vi "Set_Hi-Tec_server.vi"(4 "Client Name":string, 6 "Density Ratio":string, 7 "Strength (% by volume)":dbl min=0.0 max=5.0 format="%.3f", 8 "Stack flowrate (l/min)":dbl format="%.2f", 9 "Mode":enum16{"Control Hi-Tec", "Check Hi-Tec Demands"}(ring)) -> (0 "Flowrates (kg/min)":dbl[](array[numeric]) format="%.2f", 1 "Comment":string)   [LabVIEW 2012]
uses:
  ADAM Client/Sub VIs/ADAM Controls/Update_scan_value.ctl
  ADAM Client/Sub VIs/ADAM Controls/Ch_description_ADAM.ctl
  ADAM Client/Sub VIs/ADAM Controls/Module_type_ADAM.ctl
  ADAM Client/Sub VIs/ADAM Controls/Function_ADAM.ctl
  ADAM Client/Sub VIs/ADAM Controls/Channel_State.ctl
  ADAM Client/Sub VIs/ADAM Controls/Calib_type_ADAM.ctl
  ADAM Client/Sub VIs/ADAM Controls/Address.ctl
  Anemometry/Anemometry Sub Vis/Globals/Gas_management_global.vi
panel:
  # "-Carrier 1 only\n-Carrier 2 only\n-Enter Ratio"
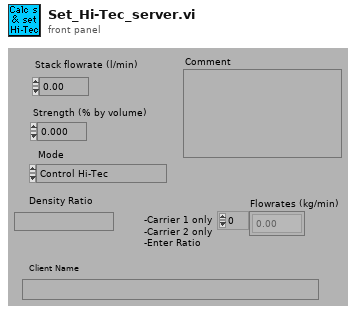
[diagram p1: front panel]
types:
  T1 = enum16{"Append to Global", "Read Global then Clear"}
  T2 = typedef "Calib_type_ADAM.ctl" = enum16{"Raw", "Bx + A", "Cx^2 + Bx + A", "Dx^3 + Cx^2 + Bx + A", "In Band", "Hi-Tec Q", "Hi-Tec M_dot", "Text"}
  T3 = typedef "Module_type_ADAM.ctl" = string
  T4 = typedef "Update_scan_value.ctl" = cluster{"Channel Name":string, "New Value":dbl}
  T5 = typedef "Ch_description_ADAM.ctl" = cluster{"Ch Name":string, "Type":T3, "Function":T6, "Ch State":T7, "Calibration type":T2, "A":dbl, "B":dbl, "C":dbl, "D":dbl, "Comments":string, "Address":T8, "String":string, "Duty":u16}
  T6 = typedef "Function_ADAM.ctl" = enum16{"Analogue Input", "Digital Input", "Event counter", "Event rate", "Analogue Output", "Digital Output", "Relay Output"}
  T7 = typedef "Channel_State.ctl" = enum16{"On", "Off", "Always On", "Always Off"}
  T8 = typedef "Address.ctl" = cluster{"Main":i32, "Ch.":i32, "Sub":i32, "Port Name":string}
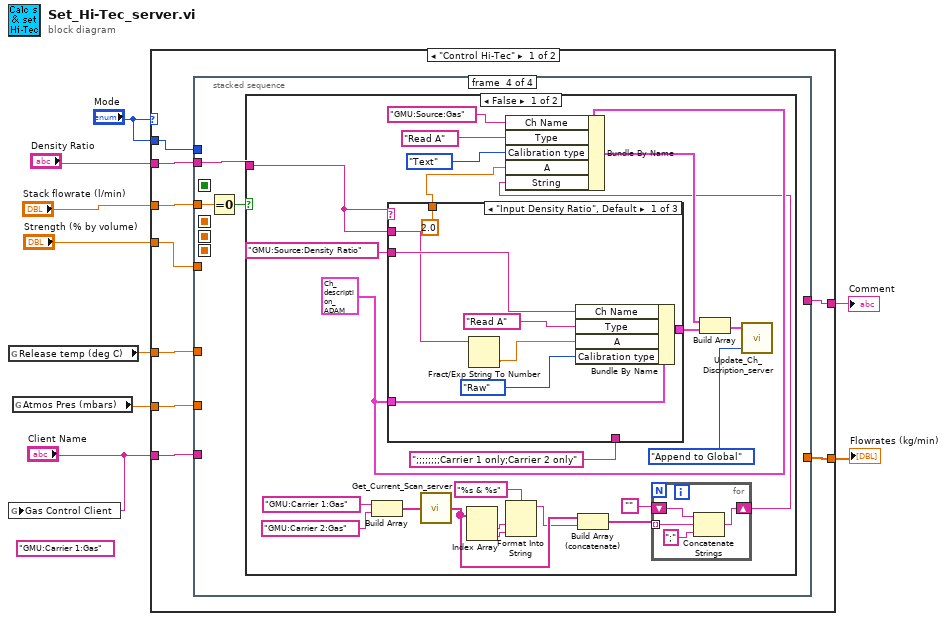
[diagram p0: block diagram]
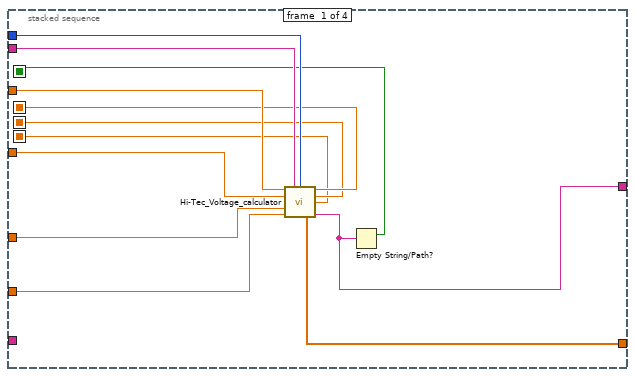
[diagram p2: hidden frame]
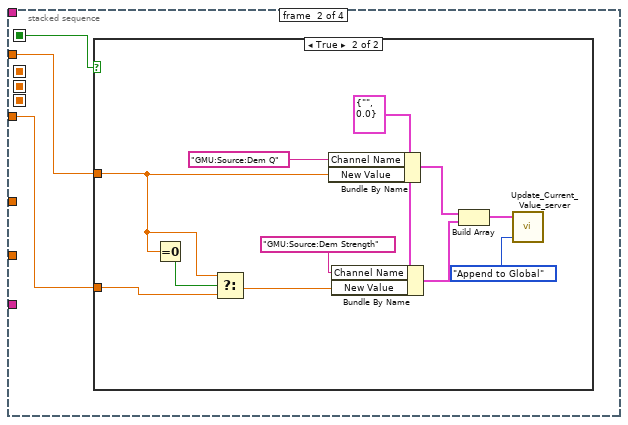
[diagram p3: hidden frame]
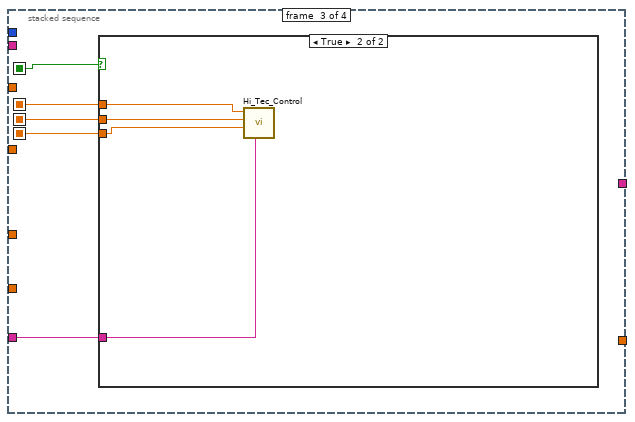
[diagram p5: hidden frame]
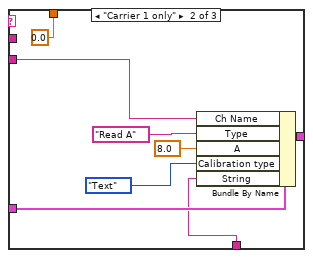
[diagram p7: hidden frame]
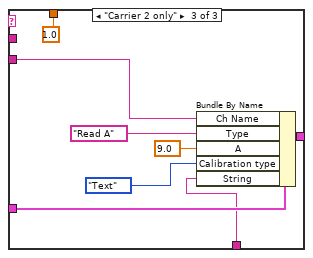
[diagram p8: hidden frame]
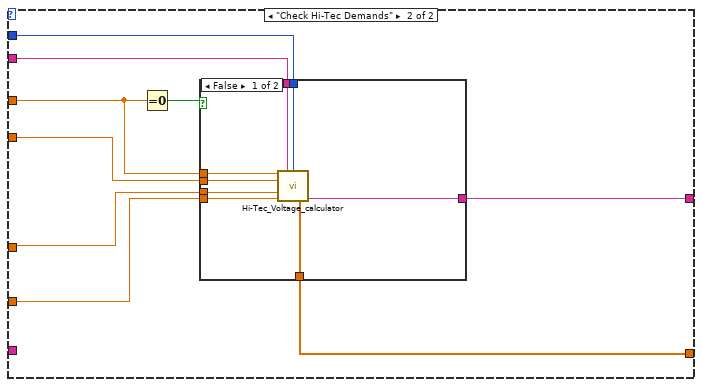
[diagram p10: hidden frame]
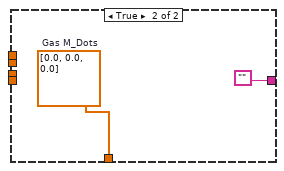
[diagram p11: hidden frame]
diagram:
  (unwired) "GMU:Carrier 1:Gas"
  n1 = global read "Gas_management_global.vi" "Release temp (deg C)"() -> (w5:dbl)
  n2 = global write "Gas_management_global.vi" "Gas Control Client"("Client Name") -> ()
  n3 = global read "Gas_management_global.vi" "Atmos Pres (mbars)"() -> (w7:dbl)
  n4 = case shown="\"Control Hi-Tec\"" "Mode" {
    tunnel: "Density Ratio" -> [w18 w113]
    tunnel: "Strength (% by volume)" -> [w17 w116]
    tunnel: "Stack flowrate (l/min)" -> [w16 w111]
    tunnel: w5 -> [w15 w115]
    tunnel: w7 -> [w14 w114]
    tunnel: [w13 w112] -> w6
    tunnel: [w12 w109] -> w3
    tunnel: "Mode" -> [w11 w108]
    tunnel: "Client Name" -> [w10 _]
    frame "Control Hi-Tec" {
      n5 = stacked-sequence {
        seq-local: [w22 _ _ _] -> [_ w31 w45 _]
        seq-local: [w21 _ _ _] -> [_ _ w49 _]
        seq-local: [w20 _ _ _] -> [_ _ w48 _]
        seq-local: [w19 _ _ _] -> [_ _ w47 _]
        tunnel: w18 -> [w28 _ _ w56]
        tunnel: w17 -> [w27 w32 _ _]
        tunnel: w16 -> [w26 w33 _ w55]
        tunnel: w15 -> [w30 _ _ _]
        tunnel: w14 -> [w29 _ _ _]
        tunnel: [w23 _ _ _] -> w13
        tunnel: [w25 _ _ _] -> w12
        tunnel: w11 -> [w24 _ _ _]
        tunnel: w10 -> [_ _ w46 _]
        frame #0 {
          n6 = call "Hi-Tec_Voltage_calculator.vi"("Stack Flowrate (l/min)"=w26, "Density Ratio"=w28, "Mode"=w24, "Strength (% by volume)"=w27, "Release temp (deg C)"=w30, "Atmos Pres (mbars)"=w29) -> ("Carrier 1 Voltage"=w21:dbl, "Carrier 2 Voltage"=w20:dbl, "Trace Voltage"=w19:dbl, "Flowrates (kg/min)"=w25:dbl[], "Error Comments"=w23:string)  [unwired: 2 in, 3 out]
          n7 = Empty String/Path?(string/path=w23) -> (empty?=w22:bool)
        }
        frame #1 {
          n8 = case shown="True" w31 {
            tunnel: w33 -> [_ w44]
            tunnel: w32 -> [_ w43]
            frame False {
            }
            frame True {
              w38 = T4 {"Channel Name"="", "New Value"=0.0} ("Update Scan Value Cluster")
              n9 = Equal To 0?(x=w44) -> (x = 0?=w35:bool)
              n10 = Select(t=w44, s=w35, f=w43) -> (s? t:f=w34:dbl)
              n11 = Bundle By Name(cluster=w38, "Channel Name"="GMU:Source:Dem Q", "New Value"=w44) -> (w41:T4)
              n12 = Bundle By Name(cluster=w38, "Channel Name"="GMU:Source:Dem Strength", "New Value"=w34) -> (w42:T4)
              n13 = Build Array(w41, w42) -> (w37:T4[])
              n14 = call "Update_Current_Value_server.vi"("Mode"=T1."Append to Global", "Update array in"=w37) -> ()  [unwired: 1 in, 1 out]
            }
          }
        }
        frame #2 {
          n15 = case shown="True" w45 {
            tunnel: w49 -> [_ w53]
            tunnel: w48 -> [_ w52]
            tunnel: w47 -> [_ w51]
            tunnel: w46 -> [_ w50]
            frame False {
            }
            frame True {
              n16 = call "Hi_Tec_Control.vi"("Carrier 1 Voltage"=w53, "Carrier 2 Voltage"=w52, "Trace Voltage"=w51, "Client Name"=w50) -> ()  [unwired: 3 out]
            }
          }
        }
        frame #3 {
          n17 = Equal To 0?(x=w55) -> (x = 0?=w54:bool)
          n18 = case shown="False" w54 {
            tunnel: w56 -> [w76 _]
            frame False {
              w67 = T5 {"Ch Name"="", "Type"="", "Function"=enum."Analogue Input", "Ch State"=enum."On", "Calibration type"=enum."Raw", "A"=0.0, "B"=0.0, "C"=0.0, "D"=0.0, "Comments"="", "Address"={"Main"=0, "Ch."=0, "Sub"=0, "Port Name"=""}, "String"="", "Duty"=65535} ("Ch Discription")
              n19 = Build Array("GMU:Carrier 1:Gas", "GMU:Carrier 2:Gas") -> (w75:string[])
              n20 = case shown="\"Input Density Ratio\", Default" w76 {
                tunnel: w67 -> [w91 w99 w107]
                tunnel: "GMU:Source:Density Ratio" -> [w90 w98 w106]
                tunnel: [w87 w94 w102] -> w78
                tunnel: w76 -> [w85 _ _]
                tunnel: ";;;;;;;;Carrier 1 only;Carrier 2 only" -> [_ w93 w101]
                tunnel: [2.0 ("A") 0.0 ("A") 1.0 ("A")] -> w57
                frame "Input Density Ratio", Default {
                  n21 = Fract/Exp String To Number(string=w85) -> (number=w86:dbl)  [unwired: 4 out]
                  n22 = Bundle By Name(cluster=w91, "Ch Name"=w90, "Type"=T3 "Read A", "A"=w86, "Calibration type"=Calib_type_ADAM."Raw") -> (w87:T5)
                }
                frame "Carrier 1 only" {
                  n23 = Bundle By Name(cluster=w99, "Ch Name"=w98, "Type"=T3 "Read A", "A"=8.0 ("Bundle Element"), "Calibration type"=Calib_type_ADAM."Text", "String"=w93) -> (w94:T5)
                }
                frame "Carrier 2 only" {
                  n24 = Bundle By Name(cluster=w107, "Ch Name"=w106, "Type"=T3 "Read A", "A"=9.0 ("Bundle Element"), "Calibration type"=Calib_type_ADAM."Text", "String"=w101) -> (w102:T5)
                }
              }
              n25 = call "Get_Current_Scan_server.vi"("Desired Channels"=w75) -> ("String values"=w63:string[])  [unwired: 2 out]
              n26 = Index Array(array=w63) -> (element #1=w66:string, element #2=w65:string)  [unwired: 2 in]
              n27 = Format Into String(format string="%s & %s", w66, w65) -> (resulting string=w62:string)  [unwired: 2 in, 1 out]
              n28 = Build Array (concatenate)(w63, w62) -> (w61:string[])
              n29 = for {
                shift-right: [w83] -> w58
                shift-left: "" -> [w82]
                tunnel: w61 -> [w81] mode=indexing
                n30 = Concatenate Strings(w82, w81, ";" ("string")) -> (w83:string)
              }
              n31 = Bundle By Name(cluster=w67, "Ch Name"="GMU:Source:Gas", "Type"=T3 "Read A", "Calibration type"=Calib_type_ADAM."Text", "A"=w57, "String"=w58) -> (w68:T5)
              n32 = Build Array(w68, w78) -> (w77:T5[])
              n33 = call "Update_Ch_Discription_server.vi"("Mode"=T1."Append to Global", "Channels to update In"=w77) -> ()  [unwired: 1 in, 1 out]
            }
            frame True {
            }
          }
        }
      }
    }
    frame "Check Hi-Tec Demands" {
      n34 = Equal To 0?(x=w111) -> (x = 0?=w110:bool)
      n35 = case shown="False" w110 {
        tunnel: w116 -> [w124 _]
        tunnel: w115 -> [w123 _]
        tunnel: w114 -> [w122 _]
        tunnel: w113 -> [w121 _]
        tunnel: [w120 ""] -> w112
        tunnel: w111 -> [w119 _]
        tunnel: [w118 w125] -> w109
        tunnel: w108 -> [w117 _]
        frame False {
          n36 = call "Hi-Tec_Voltage_calculator.vi"("Stack Flowrate (l/min)"=w119, "Density Ratio"=w121, "Mode"=w117, "Strength (% by volume)"=w124, "Release temp (deg C)"=w123, "Atmos Pres (mbars)"=w122) -> ("Flowrates (kg/min)"=w118:dbl[], "Error Comments"=w120:string)  [unwired: 1 in, 7 out]
        }
        frame True {
          w125 = dbl[] [0.0, 0.0, 0.0]  # Gas M_Dots
        }
      }
    }
  }
  "Comment" <- w6
  "Flowrates (kg/min)" <- w3
